vi "pigeon_ver4_1.vi"() -> ()   [LabVIEW 2016]
uses:
  <vilib>/Platform/TimedLoop/XDataNode/timing_clust.ctl
  <vilib>/Platform/TimedLoop/XDataNode/nitl_modes.ctl
  <vilib>/Platform/TimedLoop/XDataNode/wakeup.ctl
  <vilib>/rvi/Emulation/niFpgaGetClockAttributes.vi
  <vilib>/rvi/Emulation/niFpgaSctlEmulationGetInTimedLoop.vi
  <vilib>/rvi/Emulation/niFpgaEmulationReportErrorSimple.vi
  <vilib>/rvi/eio/common/nirviEmuTemplateMethod_errors.vi
  <vilib>/rvi/Emulation/niFpgaProcessEmulError.vi
  <vilib>/rvi/Emulation/niFpgaCriticalErrorInLSC.vi
  <vilib>/rvi/Memory/Memory_Emulation/nirvimemoryFastEmulation.vi
  <vilib>/rvi/Memory/Memory_Emulation/nirvimemoryEmulation.vi
  <vilib>/rvi/Emulation/niFpgaEmulationIsFPGAContextNoSignature.vi
  <vilib>/rvi/DataTransferAndStorage/Container/Common/niFpgaContainerGetUniqueNameForEmu.vi
  <vilib>/rvi/errors/nirviReportUnexpectedCaseInternalError (U32).vi
  <vilib>/rvi/interface/RandomDataEmulation/niFpgaRandomDataHandleErrors.vi
  <vilib>/eio/EIONode/EIONode.xnode
  <vilib>/Platform/TimedLoop/XDataNode/XDataNode.xnode
  <vilib>/rvi/DataTransferAndStorage/Container/XNode/niFpgaContainer.xnode
  <vilib>/rvi/interface/RandomDataEmulation/nirviRandomDataFpgaReadWriteTemplate.vi
  <vilib>/Platform/TimedLoop/XDataNode/XDNodeRunTimeDep.lvlib
panel:
  in  "AO5":i16
  out "AI2":i16
  in  "Tab Control":enum32{"pigeon"}(tab)
  out "trigger AI1":bool
  in  "Tab Control 2":enum32{"square wave generator 1", "coils"}(tab)
  in  "square wave  on?":bool
  in  "square wave period":i32
  in  "IGBTswitch":bool caption="IGBT Switch circular"
  in  "Manual Override":bool
  in  "circular coil current":i16(slide) scale=0.0..32768.0
  out "FIFO size":i16
  in  "AO0":i16
  in  "AO1":i16
  in  "AO2":i16
  in  "Run program":bool
  in  "halt processor":bool
  out "control flags":i8 format="%b"
  in  "host operation":i16
  in  "address":u16
  in  "data1":u16
  in  "data2":i32
  in  "repeat program":i32
  out "IP address":i16
  out "PMT1":i16=-4740
  out "ReA":i32
  out "RegB":i16
  out "RegC":i16
  out "exttrigger":bool=TRUE
  out "AI1":i16=161
  out "RegD":i16
  in  "AO4":i16
  in  "AO3":i16
  out "Connector0/AI0":i16
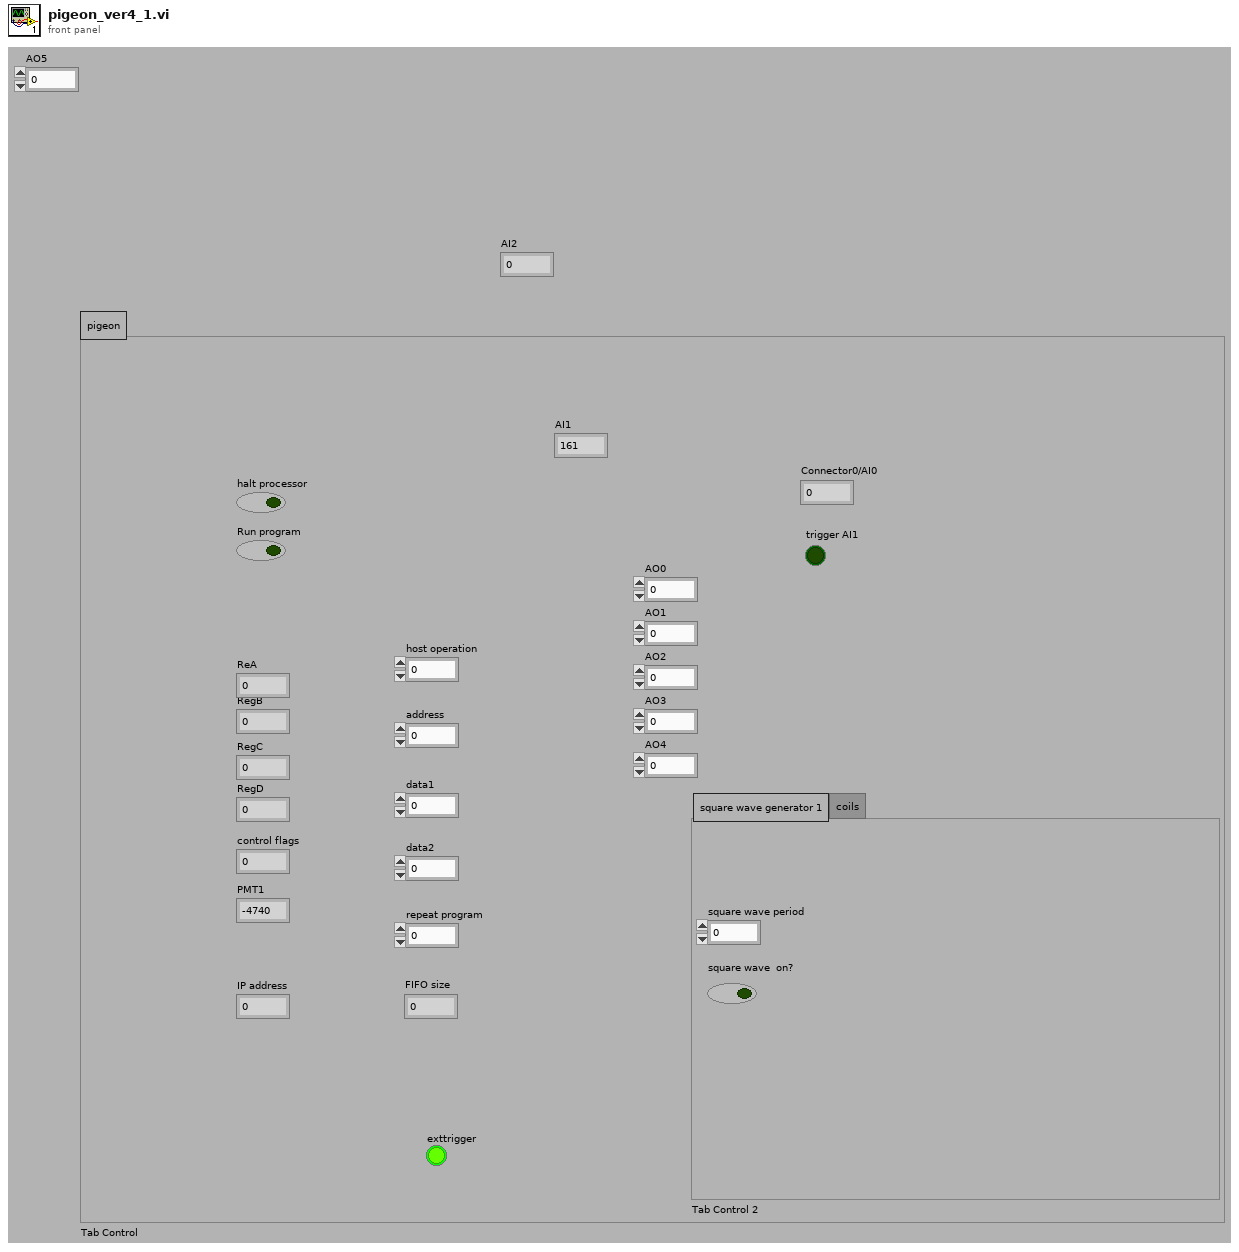
[diagram p1: front panel]
types:
  T1 = typedef "XDNodeRunTimeDep.lvlib/timing_clust.ctl" = cluster{"Expected End [f-1]":u64, "Actual End [f-1]":u64, "Finished Late? [f-1]":bool, "Expected End [i-1]":u64, "Actual End [i-1]":u64, "Finished Late? [i-1]":bool, "Expected Start [i]":u64, "Actual Start [i]":u64, "Expected Start [f]":u64, "Actual Start [f]":u64, "Source Name":string, "Structure Name":string, "Period":i64, "Deadline":i64, "Offset":i64, "Start":i64, "Priority":i32, "Timeout":i32, "Mode":T2, "Wakeup Reason":T3, "Error":errorcluster, "Source Type":string, "Secondary Source Type":string, "Global End Time":u64, "Global Start Time":u64, "Frame Duration":u64, "Iteration Duration":u64, "Assigned CPU":i32, "I/O Scan Engine Mode":u32}
  T2 = typedef "XDNodeRunTimeDep.lvlib/nitl_modes.ctl" = enum32{"No Change", "Process missed periods, maintain original phase", "Discard missed periods, maintain original phase", "Process missed periods, ignore original phase", "Discard missed periods, ignore original phase"}
  T3 = typedef "XDNodeRunTimeDep.lvlib/wakeup.ctl" = enum32{"Normal", "Aborted", "Asynchronous wakeup", "Timing source error", "Timed loop error", "Timeout"}
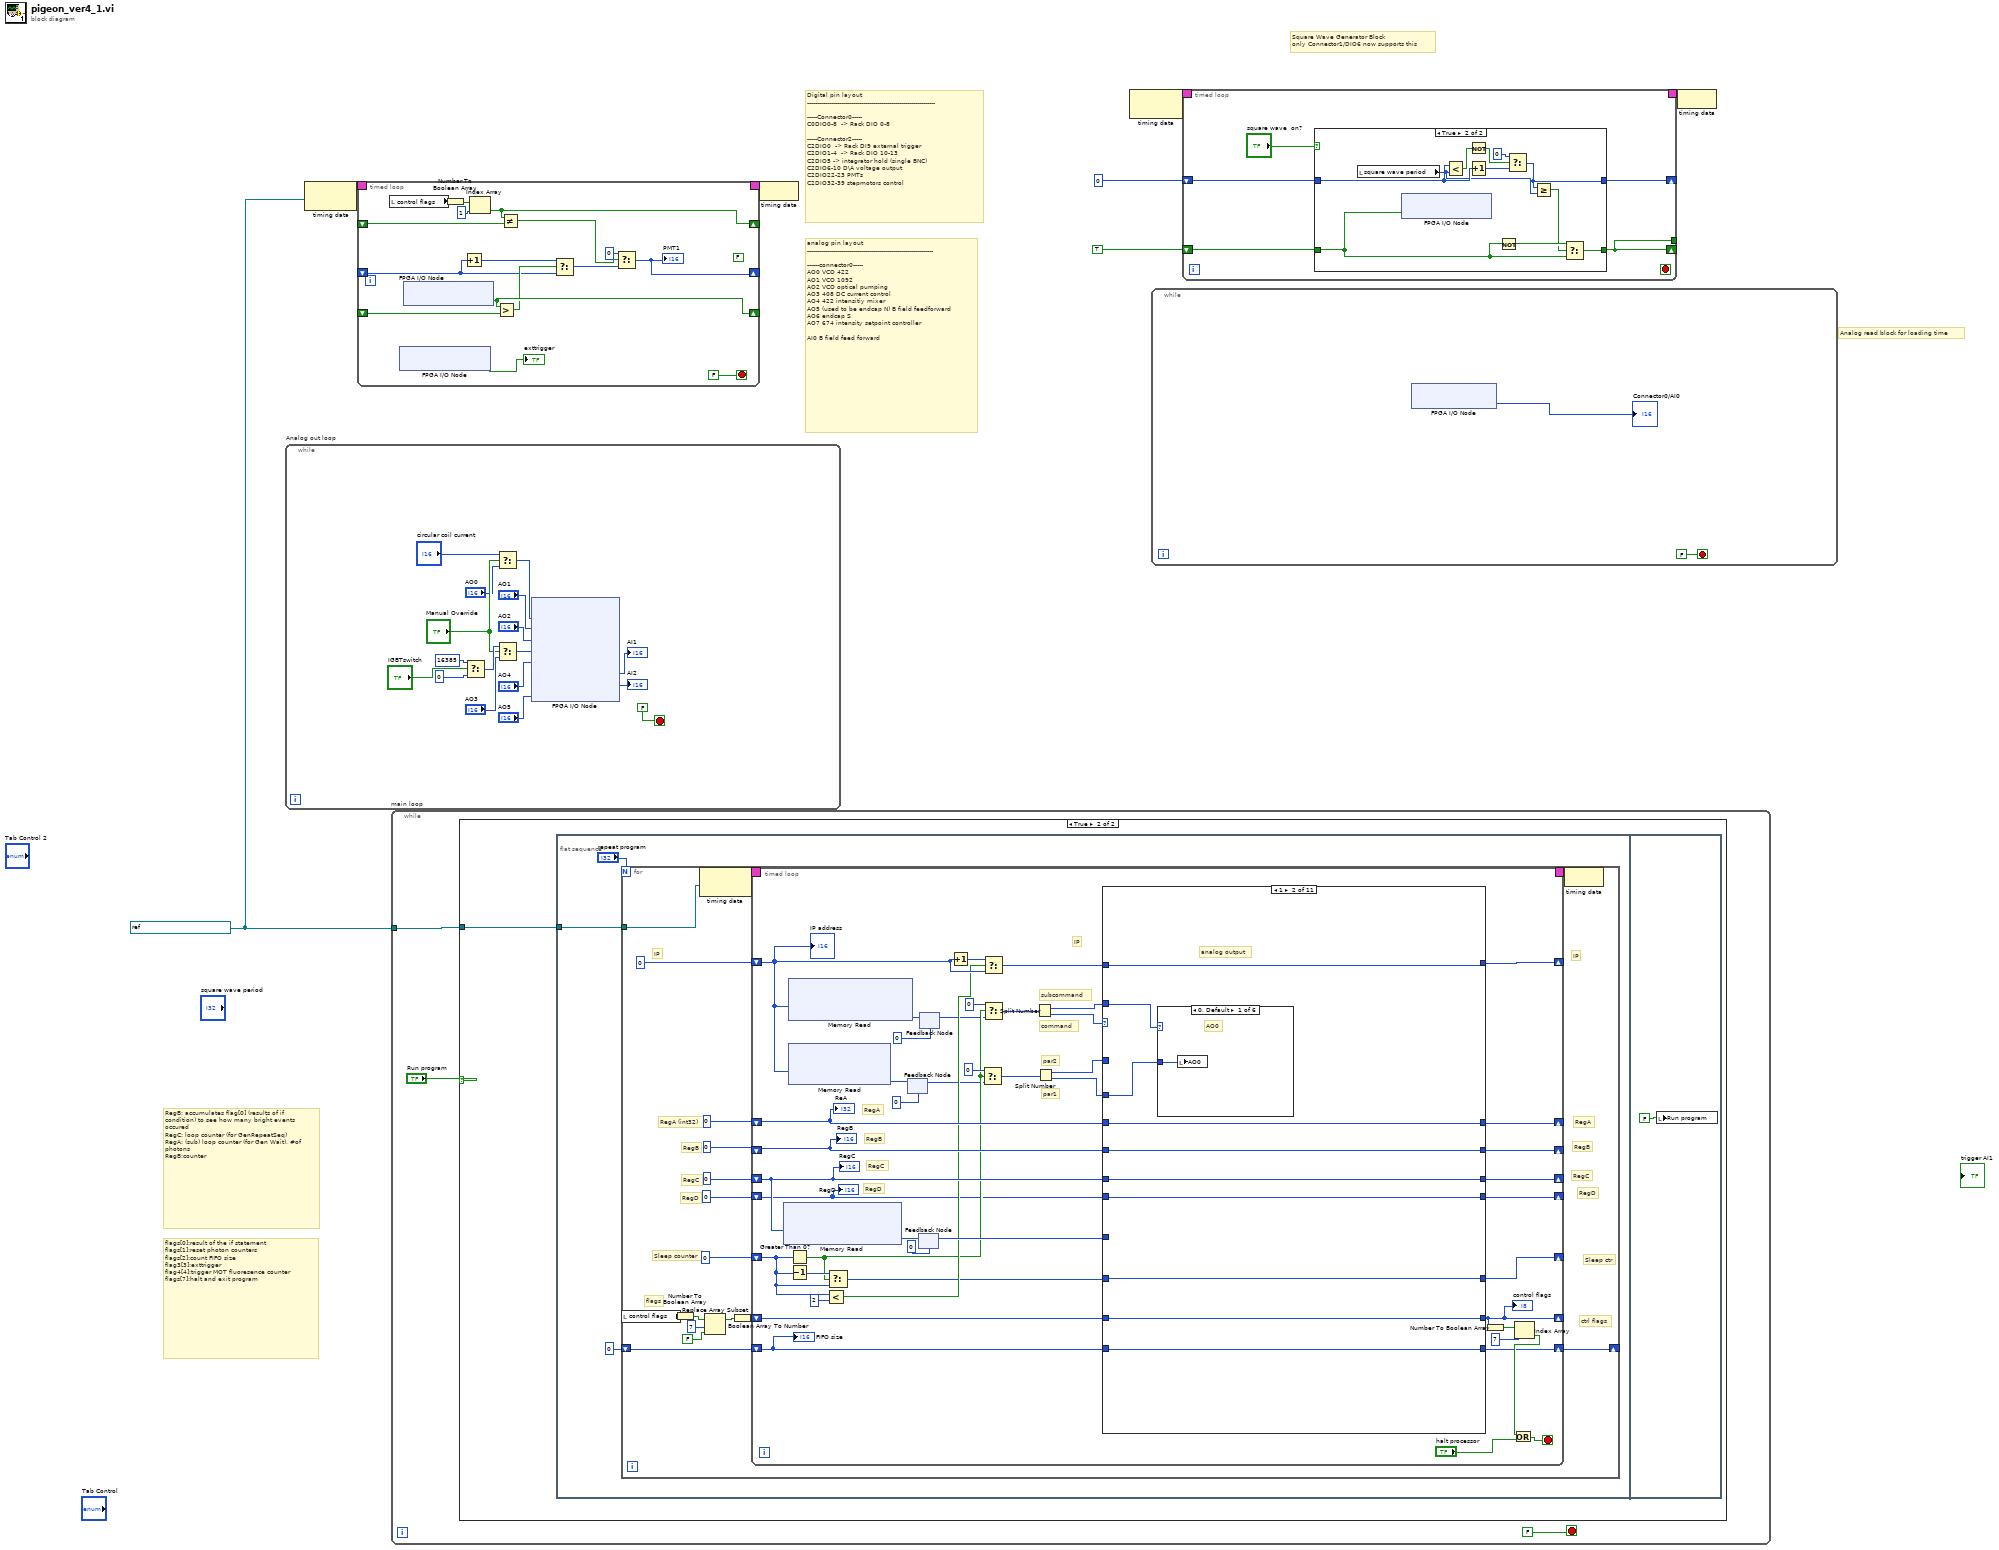
[diagram p0: block diagram]
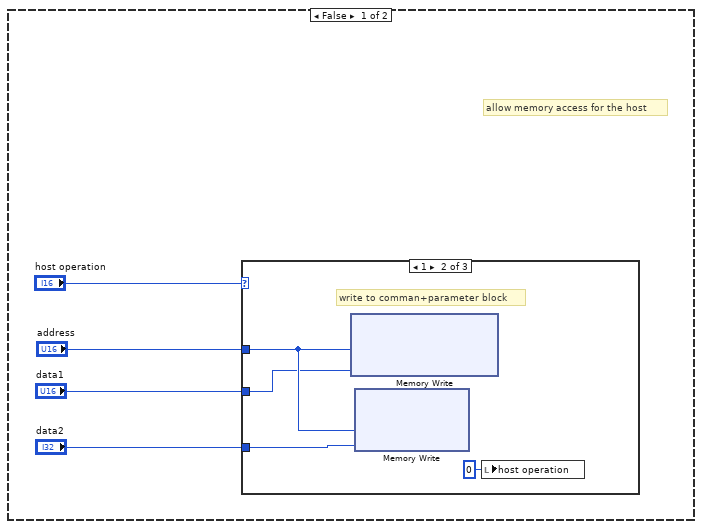
[diagram p3: hidden frame]
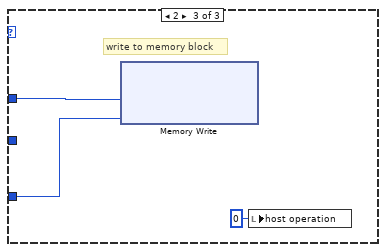
[diagram p5: hidden frame]
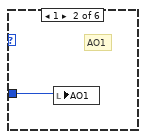
[diagram p7: hidden frame]
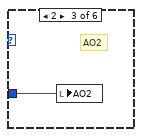
[diagram p8: hidden frame]
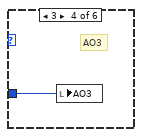
[diagram p9: hidden frame]
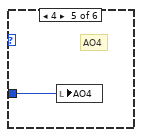
[diagram p10: hidden frame]
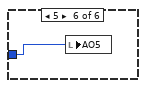
[diagram p11: hidden frame]
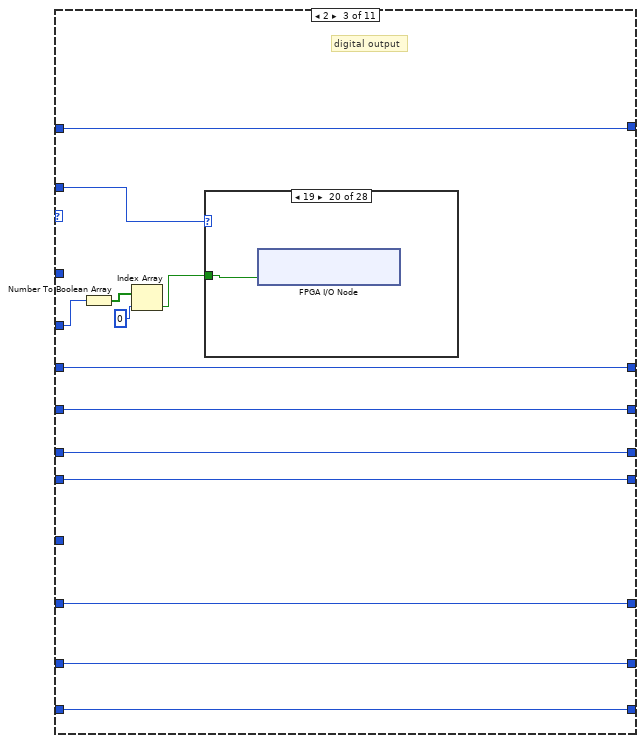
[diagram p12: hidden frame]
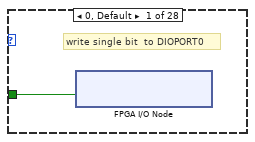
[diagram p13: hidden frame]
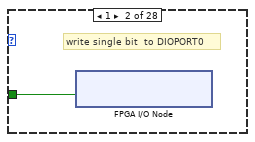
[diagram p14: hidden frame]
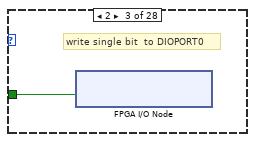
[diagram p15: hidden frame]
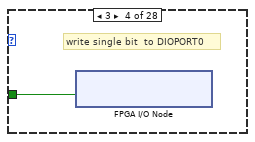
[diagram p16: hidden frame]
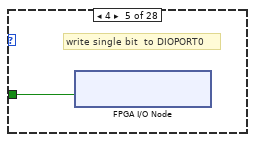
[diagram p17: hidden frame]
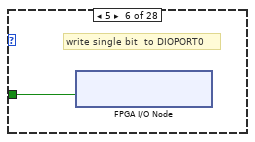
[diagram p18: hidden frame]
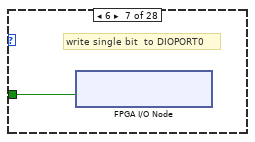
[diagram p19: hidden frame]
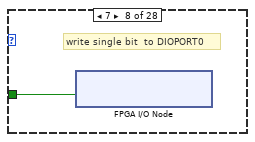
[diagram p20: hidden frame]
diagram:
  w5 = refnum<k21> "40 MHz Onboard Clock" ("FPGA Clock")
  # "Analog read block for loading time"
  # "Square Wave Generator Block\nonly Connector1/DIO6 now supports this"
  # "RegB: accumulates flag[0] (results of if condition) to see how many bright events occured\nRegC: loop counter (for GenRepeatSeq)\nRegA: (sub) loop counter (for Gen Wait), #of     photons \nRegB:counter"
  # "flags[0]:result of the if statement\nflags[1]:reset photon counters\nflags[2]:count FIFO size\nflag3[3]:exttrigger\nflag4[4]:trigger MOT fluoresence counter\nflags[7]:halt and exit program"
  # "Digital pin layout\n----------------------------------------------------------------\n\n-----Connector0-----\nC0DIO0-8  -> Rack DIO 0-8\n\n-----Connector2-----\nC2DIO0  -> Rack DI9 external trigger \nC2DIO1-4  -> Rack DIO 10-13\nC2DIO5 -> integrator hold (single BNC)\nC2DIO6-10 D\\A voltage output\nC2DIO22-23 PMTs\nC2DIO32-39 stepmotors control"
  # "analog pin layout\n---------------------------------------------------------------\n\n------connector0-----\nAO0 VCO 422\nAO1 VCO 1092\nAO2 VCO optical pumping\nAO3 408 DC current control\nAO4 422 intensitiy mixer\nAO5 (used to be endcap N) B field feedforward\nAO6 endcap S\nAO7 674 intensity setpoint controller\n\nAI0 B field feed forward"
  n1 = while "Analog out loop" {
    stop <- FALSE stop-if-true
    n2 = Select(t=i16 16385, s="IGBTswitch", f=i16 0) -> (s? t:f=w14:i16)
    n3 = Select(t="circular coil current", s="Manual Override", f="AO0") -> (s? t:f=w8:i16)
    n4 = Select(t=w14, s="Manual Override", f="AO3") -> (s? t:f=w13:i16)
    n5 = xnode "FPGA I/O Node"("Connector0/AO0"=w8, "Connector0/AO1"="AO1", "Connector0/AO2"="AO2", "Connector0/AO3"=w13, "Connector0/AO4"="AO4", "Connector0/AO5"="AO5") -> ("Connector0/AI1"=→"AI1":i16, "Connector0/AI2"=→"AI2":i16)  [unwired: 8 in, 8 out]
  }
  n6 = node-c288(w5) -> (w7:T1)
  n7 = timed-loop {
    timing: w7 -> [_]
    timing-out: [_] -> w6
    shift-right: [w38] -> _
    shift-left: _ -> [w27]
    shift-right: [w31] -> _
    shift-left: _ -> [w40]
    shift-right: [w33] -> _
    shift-left: _ -> [w34]
    stop <- FALSE stop-if-true
    (unwired) FALSE
    n8 = local read "control flags"() -> (w35:i8)
    n9 = xnode "FPGA I/O Node"() -> ("Connector2/DIO0"=→"exttrigger":bool)  [unwired: 1 in, 1 out]
    n10 = xnode "FPGA I/O Node"() -> ("Connector0/DIO0"=w31:bool)  [unwired: 1 in, 1 out]
    n11 = Number To Boolean Array(number=w35) -> (Boolean array=w36:bool[])
    n12 = Increment(x=w27) -> (x+1=w28:u16)
    n13 = Index Array(array=w36, index=1) -> (element=w33:bool)
    n14 = Greater?(x=w31, y=w40) -> (0:w30:bool)
    n15 = Not Equal?(x=w33, y=w34) -> (x != y?=w25:bool)
    n16 = Select(t=w28, s=w30, f=w27) -> (s? t:f=w39:u16)
    n17 = Select(t=u16 0, s=w25, f=w39) -> (s? t:f=w38:u16)
    "PMT1" <- w38
  }
  n18 = while "main loop" {
    tunnel: w5 -> [w43]
    stop <- FALSE ("stop") stop-if-true
    n19 = case shown="True" "Run program" {
      tunnel: w43 -> [_ w57]
      frame False {
        # "allow memory access for the host"
        n20 = case shown="1" "host operation" {
          tunnel: "address" -> [_ w51 w56]
          tunnel: "data1" -> [_ w50 _]
          tunnel: "data2" -> [_ w53 w54]
          frame 0, Default {
          }
          frame 1 {
            # "write to comman+parameter block"
            n21 = xnode ("Memory Write")("Address"=w51, "Data"=w50) -> ()  [unwired: 1 in, 1 out]
            n22 = xnode ("Memory Write")("Address"=w51, "Data"=w53) -> ()  [unwired: 1 in, 1 out]
            n23 = local write "host operation"(i16 0 ("host operation")) -> ()
          }
          frame 2 {
            # "write to memory block"
            n24 = xnode ("Memory Write")("Address"=w56, "Data"=w54) -> ()  [unwired: 1 in, 1 out]
            n25 = local write "host operation"(i16 0 ("host operation")) -> ()
          }
        }
      }
      frame True {
        n26 = flat-sequence {
          tunnel: w57 -> [w59]
          frame #0 {
            n27 = for {
              N: "repeat program" -> [_]
              tunnel: w59 -> [w71]
              shift-right: [w62] -> _
              shift-left: i16 0 -> [w63]
              # "ctrl flags"
              # "Sleep ctr"
              # "RegD"
              # "RegD"
              # "Sleep counter"
              # "flags"
              # "RegC"
              # "RegB"
              # "RegA"
              # "RegC"
              # "RegB"
              # "RegA (int32)"
              # "IP"
              # "IP"
              n28 = local read "control flags"() -> (w66:i8)
              n29 = Number To Boolean Array(number=w66) -> (Boolean array=w70:bool[])
              n30 = node-c288(w71) -> (w77:T1)
              n31 = Replace Array Subset(array=w70, new element=FALSE ("new element/subarray"), index=7) -> (w68:bool[])
              n32 = Boolean Array To Number(Boolean array=w68) -> (number=w69:u8)
              n33 = timed-loop {
                timing: w77 -> [_]
                timing-out: [_] -> w76
                shift-right: [w112] -> _
                shift-left: i16 0 -> [w95]
                shift-right: [w108] -> _
                shift-left: 0 -> [w104]
                shift-right: [w120] -> _
                shift-left: i16 0 -> [w111]
                shift-right: [w119] -> _
                shift-left: i16 0 -> [w103]
                shift-right: [w109] -> _
                shift-left: w69 -> [w110]
                shift-right: [w102] -> _
                shift-left: i16 0 -> [w93]
                shift-right: [w84] -> w62
                shift-left: w63 -> [w83]
                shift-right: [w81] -> _
                shift-left: i16 0 -> [w82]
                stop <- w115 stop-if-true
                # "RegD"
                # "IP"
                # "RegC"
                # "RegB"
                # "RegA"
                # "par1"
                # "par2"
                # "subcommand"
                # "command"
                n34 = xnode ("Memory Read")("Address"=w103) -> ("Data"=w107:i16)  [unwired: 2 in, 2 out]
                n35 = xnode ("Memory Read")("Address"=w95) -> ("Data"=w90:u16)  [unwired: 1 in, 1 out]
                n36 = xnode ("Memory Read")("Address"=w95) -> ("Data"=w86:i32)  [unwired: 1 in, 1 out]
                n37 = Greater Than 0?(x=w93) -> (x > 0?=w88:bool)
                n38 = Decrement(x=w93) -> (x-1=w94:u32)
                n39 = Less?(x=w93, y=u32 2) -> (x < y?=w92:bool)
                n40 = Select(t=w94, s=w88, f=w93) -> (s? t:f=w91:u32)
                n41 = feedback-in #1(w86) -> ()
                n42 = feedback #1(u32 0 ("Data")) -> (w85:u32)
                n43 = feedback-in #2(w107) -> ()
                n44 = feedback #2(0) -> (w106:i32)
                n45 = feedback-in #3(w90) -> ()
                n46 = feedback #3(u16 0 ("Data")) -> (w87:u16)
                n47 = Increment(x=w95) -> (x+1=w96:u16)
                n48 = Select(t=0, s=w88, f=w85) -> (s? t:f=w99:u32)
                n49 = Select(t=w96, s=w92, f=w95) -> (s? t:f=w101:u16)
                n50 = Select(t=u16 0, s=w88, f=w87) -> (s? t:f=w100:u16)
                n51 = Split Number(x=w100) -> (hi(x)=w121:u8, lo(x)=w122:u8)
                n52 = Split Number(x=w99) -> (hi(x)=w113:u16, lo(x)=w114:u16)
                n53 = case shown="1" w122 {
                  tunnel: w114 -> [_ w139 w151 _ w231 w351 w425 _ _ w484 _]
                  tunnel: w113 -> [_ _ _ _ w224 w350 w424 _ _ w485 _]
                  tunnel: w121 -> [_ w140 w159 w198 w232 w355 _ w443 _ w467 _]
                  tunnel: w104 -> [w130 w138 w158 w190 w230 w352 w429 w447 w463 w483 w502]
                  tunnel: [w130 w138 w158 w190 w227 w352 w429 w447 w463 w482 w502] -> w108
                  tunnel: w111 -> [w129 w137 w157 w189 w229 w353 w430 w446 w466 w481 w503]
                  tunnel: w103 -> [w128 w136 w156 w196 w228 w354 w431 w445 w465 w479 w504]
                  tunnel: [w129 w137 w157 w188 w226 w353 w430 w446 w466 w480 w503] -> w120
                  tunnel: [w128 w136 w156 w196 w225 w354 w431 w445 w465 w478 w504] -> w119
                  tunnel: [w126 w135 w155 w197 w220 w358 w423 w449 w464 w468 w501] -> w112
                  tunnel: w101 -> [w126 w135 w155 w197 w221 w358 _ w449 w464 w469 w501]
                  tunnel: [w127 w134 w154 w194 w222 w357 w422 w438 w460 w472 w507] -> w109
                  tunnel: w110 -> [w127 w134 w154 w195 w223 w356 w422 w437 w459 w473 w507]
                  tunnel: w106 -> [_ _ _ _ w214 w349 _ _ _ _ _]
                  tunnel: w91 -> [w125 w133 w149 w193 w219 w348 w421 w435 w456 w475 w508]
                  tunnel: [w125 w133 w149 w193 w218 w348 w421 w435 w456 w474 w508] -> w102
                  tunnel: w83 -> [w124 w132 w148 w192 w217 w347 w420 w434 w455 w470 w506]
                  tunnel: [w124 w132 w148 w192 w217 w347 w420 w433 w455 w471 w506] -> w84
                  tunnel: w82 -> [w123 w131 w147 w191 w216 w346 w419 w432 w454 w477 w505]
                  tunnel: [w123 w131 w147 w191 w215 w346 w419 w432 w454 w476 w505] -> w81
                  frame 0, Default {
                  }
                  frame 1 {
                    # "analog output"
                    n54 = case shown="0, Default" w140 {
                      tunnel: w139 -> [w141 w142 w143 w144 w145 w146]
                      frame 0, Default {
                        # "AO0"
                        n55 = local write "AO0"(w141) -> ()
                      }
                      frame 1 {
                        # "AO1"
                        n56 = local write "AO1"(w142) -> ()
                      }
                      frame 2 {
                        # "AO2"
                        n57 = local write "AO2"(w143) -> ()
                      }
                      frame 3 {
                        # "AO3"
                        n58 = local write "AO3"(w144) -> ()
                      }
                      frame 4 {
                        # "AO4"
                        n59 = local write "AO4"(w145) -> ()
                      }
                      frame 5 {
                        n60 = local write "AO5"(w146) -> ()
                      }
                    }
                  }
                  frame 2 {
                    # "digital output"
                    n61 = Number To Boolean Array(number=w151) -> (Boolean array=w152:bool[])
                    n62 = Index Array(array=w152, index=0) -> (element=w150:bool)
                    n63 = case shown="19" w159 {
                      tunnel: w150 -> [w160 w161 w162 w163 w164 w165 w166 w167 w168 w169 w170 w171 w172 w173 w174 w175 w176 w177 w178 w179 w180 w181 w182 w183 w184 w185 w186 w187]
                      frame 0, Default {
                        # "write single bit  to DIOPORT0"
                        n64 = xnode "FPGA I/O Node"("Connector1/DIO0"=w160) -> ()  [unwired: 1 in, 1 out]
                      }
                      frame 1 {
                        # "write single bit  to DIOPORT0"
                        n65 = xnode "FPGA I/O Node"("Connector1/DIO1"=w161) -> ()  [unwired: 1 in, 1 out]
                      }
                      frame 2 {
                        # "write single bit  to DIOPORT0"
                        n66 = xnode "FPGA I/O Node"("Connector1/DIO2"=w162) -> ()  [unwired: 1 in, 1 out]
                      }
                      frame 3 {
                        # "write single bit  to DIOPORT0"
                        n67 = xnode "FPGA I/O Node"("Connector1/DIO3"=w163) -> ()  [unwired: 1 in, 1 out]
                      }
                      frame 4 {
                        # "write single bit  to DIOPORT0"
                        n68 = xnode "FPGA I/O Node"("Connector1/DIO4"=w164) -> ()  [unwired: 1 in, 1 out]
                      }
                      frame 5 {
                        # "write single bit  to DIOPORT0"
                        n69 = xnode "FPGA I/O Node"("Connector1/DIO5"=w165) -> ()  [unwired: 1 in, 1 out]
                      }
                      frame 6 {
                        # "write single bit  to DIOPORT0"
                        n70 = xnode "FPGA I/O Node"("Connector1/DIO6"=w166) -> ()  [unwired: 1 in, 1 out]
                      }
                      frame 7 {
                        # "write single bit  to DIOPORT0"
                        n71 = xnode "FPGA I/O Node"("Connector1/DIO7"=w167) -> ()  [unwired: 1 in, 1 out]
                      }
                      frame 8 {
                        # "write single bit  to DIOPORT0"
                        n72 = xnode "FPGA I/O Node"("Connector1/DIO8"=w168) -> ()  [unwired: 1 in, 1 out]
                      }
                      frame 9 {
                        n73 = xnode "FPGA I/O Node"("Connector1/DIO9"=w169) -> ()  [unwired: 1 in, 1 out]
                      }
                      frame 10 {
                        n74 = xnode "FPGA I/O Node"("Connector1/DIO10"=w170) -> ()  [unwired: 1 in, 1 out]
                      }
                      frame 11 {
                        n75 = xnode "FPGA I/O Node"("Connector1/DIO11"=w171) -> ()  [unwired: 1 in, 1 out]
                      }
                      frame 12 {
                        n76 = xnode "FPGA I/O Node"("Connector1/DIO12"=w172) -> ()  [unwired: 1 in, 1 out]
                      }
                      frame 13 {
                        n77 = xnode "FPGA I/O Node"("Connector1/DIO13"=w173) -> ()  [unwired: 1 in, 1 out]
                      }
                      frame 14 {
                        n78 = xnode "FPGA I/O Node"("Connector1/DIO14"=w174) -> ()  [unwired: 1 in, 1 out]
                      }
                      frame 15 {
                        n79 = xnode "FPGA I/O Node"("Connector1/DIO15"=w175) -> ()  [unwired: 1 in, 1 out]
                      }
                      frame 16 {
                        n80 = xnode "FPGA I/O Node"("Connector1/DIO16"=w176) -> ()  [unwired: 1 in, 1 out]
                      }
                      frame 17 {
                        n81 = xnode "FPGA I/O Node"("Connector1/DIO17"=w177) -> ()  [unwired: 1 in, 1 out]
                      }
                      frame 18 {
                        n82 = xnode "FPGA I/O Node"("Connector1/DIO18"=w178) -> ()  [unwired: 1 in, 1 out]
                      }
                      frame 19 {
                        n83 = xnode "FPGA I/O Node"("Connector1/DIO19"=w179) -> ()  [unwired: 1 in, 1 out]
                      }
                      frame 20 {
                        n84 = xnode "FPGA I/O Node"("Connector2/DIO12"=w180) -> ()  [unwired: 1 in, 1 out]
                      }
                      frame 21 {
                        n85 = xnode "FPGA I/O Node"("Connector2/DIO17"=w181) -> ()  [unwired: 1 in, 1 out]
                      }
                      frame 22 {
                        n86 = xnode "FPGA I/O Node"("Connector2/DIO19"=w182) -> ()  [unwired: 1 in, 1 out]
                      }
                      frame 23 {
                        n87 = xnode "FPGA I/O Node"("Connector2/DIO18"=w183) -> ()  [unwired: 1 in, 1 out]
                      }
                      frame 24 {
                        n88 = xnode "FPGA I/O Node"("Connector2/DIO21"=w184) -> ()  [unwired: 1 in, 1 out]
                      }
                      frame 25 {
                        n89 = xnode "FPGA I/O Node"("Connector2/DIO24"=w185) -> ()  [unwired: 1 in, 1 out]
                      }
                      frame 26 {
                        n90 = xnode "FPGA I/O Node"("Connector2/DIO25"=w186) -> ()  [unwired: 1 in, 1 out]
                      }
                      frame 27 {
                        n91 = xnode "FPGA I/O Node"("Connector2/DIO20"=w187) -> ()  [unwired: 1 in, 1 out]
                      }
                    }
                  }
                  frame 3 {
                    # "photon counting"
                    n92 = case shown="3" w198 {
                      tunnel: [w199 w201 w213] -> w188
                      tunnel: w189 -> [w199 w202 w213]
                      tunnel: w195 -> [w200 w204 w211]
                      tunnel: [w200 w204 w210] -> w194
                      frame 2, Default {
                      }
                      frame 1 {
                        # "PMT1"
                        n93 = local read "PMT1"() -> (w203:i16)
                        n94 = Add(x=w203, y=w202) -> (x+y=w201:u16)
                      }
                      frame 3 {
                        # "Reset  photon counter"
                        # "make a Not gate of flag(1)"
                        n95 = Number To Boolean Array(number=w211) -> (Boolean array=w208:bool[])
                        n96 = Index Array(array=w208, index=1) -> (element=w206:bool)
                        n97 = Not(x=w206) -> (.not. x?=w205:bool)
                        n98 = Replace Array Subset(array=w208, new element=w205, index=1) -> (w209:bool[])
                        n99 = Boolean Array To Number(Boolean array=w209) -> (number=w210:u8)
                      }
                    }
                  }
                  frame 4 {
                    # "registers operation"
                    n100 = case shown="7" w232 {
                      tunnel: w231 -> [w238 w248 w255 _ _ _ _ w297 _ _ w324 w337]
                      tunnel: w230 -> [_ w247 w254 w261 w269 w277 w281 w302 w313 w319 w329 w342]
                      tunnel: w229 -> [w241 _ w253 w260 w271 w276 w289 w301 w312 w315 w327 w340]
                      tunnel: w228 -> [w240 w246 _ w263 w270 _ w282 w300 w311 w318 w328 w341]
                      tunnel: [w237 w247 w254 w261 w268 w277 w281 w302 w313 w319 w329 w342] -> w227
                      tunnel: [w241 w248 w253 w260 w271 w276 w288 w301 w312 w317 w327 w340] -> w226
                      tunnel: [w240 w246 w255 w262 w270 w276 w282 w300 w311 w318 w328 w341] -> w225
                      tunnel: w224 -> [w239 _ _ _ _ _ _ w298 _ _ _ w336]
                      tunnel: w223 -> [w236 w245 w252 w259 w267 w275 w283 w299 w310 w322 w332 w345]
                      tunnel: [w236 w245 w252 w259 w267 w275 w283 w299 w310 w322 w332 w345] -> w222
                      tunnel: w221 -> [w235 w244 w251 w258 w266 w274 w280 w291 w305 w321 w331 w344]
                      tunnel: [w235 w244 w251 w258 w266 w274 w280 w294 w308 w321 w331 w344] -> w220
                      tunnel: w219 -> [w234 w243 w250 w257 w265 w273 w279 _ _ w320 w330 w343]
                      tunnel: [w234 w243 w250 w257 w265 w273 w279 w295 w303 w320 w330 w343] -> w218
                      tunnel: w216 -> [w233 w242 w249 w256 w264 w272 w278 w290 w304 w314 _ w335]
                      tunnel: [w233 w242 w249 w256 w264 w272 w278 w290 w304 w314 w325 w334] -> w215
                      tunnel: w214 -> [_ _ _ _ _ _ _ _ w303 _ _ _]
                      frame 0, Default {
                        # "Set par1,2 to RegA"
                        n101 = Join Numbers(hi=w239, lo=w238) -> ((hi.lo)=w237:u32)
                      }
                      frame 1 {
                        # "Set par1 to RegB"
                      }
                      frame 2 {
                        # "Set par1 to RegC"
                      }
                      frame 3 {
                        # "increase RegC by 1"
                        n102 = Increment(x=w263) -> (x+1=w262:u16)
                      }
                      frame 4 {
                        # "increase RegA by 1"
                        n103 = Increment(x=w269) -> (x+1=w268:u32)
                      }
                      frame 5 {
                        # "Set regC to regB"
                      }
                      frame 6 {
                        # "regB<-regB+flags[0]"
                        n104 = Number To Boolean Array(number=w283) -> (Boolean array=w287:bool[])
                        n105 = Index Array(array=w287, index=0) -> (element=w285:bool)
                        n106 = Boolean To (0,1)(Boolean=w285) -> (0, 1=w284:i16)
                        n107 = Add(x=w284, y=w289) -> (x+y=w288:u16)
                      }
                      frame 7 {
                        # "Sleep counter = [par1 par2]"
                        n108 = Join Numbers(hi=w298, lo=w297) -> ((hi.lo)=w295:u32)
                        n109 = Greater?(x=w295, y=u32 0) -> (0:w293:bool)
                        n110 = Decrement(x=w291) -> (x-1=w292:u16)
                        n111 = Select(t=w292, s=w293, f=w291) -> (s? t:f=w294:u16)
                      }
                      frame 11 {
                        # "Sleep counter =par1* memory Block[RegC]"
                        n112 = Greater?(x=w303, y=u32 0) -> (0:w307:bool)
                        n113 = Decrement(x=w305) -> (x-1=w306:u16)
                        n114 = Select(t=w306, s=w307, f=w305) -> (s? t:f=w308:u16)
                      }
                      frame 8 {
                        # "RegB=RegB+ RegA(lo)"
                        n115 = Split Number(x=w319) -> (lo(x)=w316:u16)  [unwired: 1 out]
                        n116 = Add(x=w316, y=w315) -> (x+y=w317:u16)
                      }
                      frame 9 {
                        # "RegD<-AI1+par1"
                        n117 = To Word Integer(number=w324) -> (16bit integer=w323:i16)
                        n118 = local read "AI1"() -> (w326:i16)
                        n119 = Add(x=w323, y=w326) -> (x+y=w325:i16)
                      }
                      frame 10 {
                        # "RegD<-RegD*2^par1*par2"
                        n120 = To Word Integer(number=w336) -> (16bit integer=w338:i16)
                        n121 = To Word Integer(number=w337) -> (16bit integer=w339:i16)
                        n122 = Multiply(x=w338, y=w335) -> (x*y=w333:i16)
                        n123 = Scale By Power Of 2(n=w339, x=w333) -> (x*2^n=w334:i16)
                      }
                    }
                  }
                  frame 5 {
                    # "If statement"
                    n124 = case shown="4" w355 {
                      tunnel: [w368 w376 w384 w392 w402 w405 w413] -> w357
                      tunnel: w356 -> [w367 w375 w383 w391 w401 w406 w414]
                      tunnel: w350 -> [w361 _ _ _ _ _ _]
                      tunnel: w354 -> [_ _ w379 w386 _ _ _]
                      tunnel: w353 -> [_ w370 _ w385 _ _ _]
                      tunnel: w352 -> [w362 _ _ _ _ w403 w411]
                      tunnel: w351 -> [w360 w369 w378 _ _ w404 _]
                      tunnel: w349 -> [_ _ _ _ _ _ w418]
                      frame 0, Default {
                        # "The if regA =  [par1,par2]"
                        n125 = Number To Boolean Array(number=w367) -> (Boolean array=w365:bool[])
                        n126 = Join Numbers(hi=w361, lo=w360) -> ((hi.lo)=w359:u32)
                        n127 = Equal?(x=w359, y=w362) -> (x = y?=w363:bool)
                        n128 = Replace Array Subset(array=w365, new element=w363, index=0) -> (w364:bool[])
                        n129 = Boolean Array To Number(Boolean array=w364) -> (number=w368:u8)
                      }
                      frame 1 {
                        # "The if  regB >  par1"
                        n130 = Number To Boolean Array(number=w375) -> (Boolean array=w373:bool[])
                        n131 = Greater?(x=w370, y=w369) -> (0:w371:bool)
                        n132 = Replace Array Subset(array=w373, new element=w371, index=0) -> (w372:bool[])
                        n133 = Boolean Array To Number(Boolean array=w372) -> (number=w376:u8)
                      }
                      frame 2 {
                        # "The if  regC=  par1"
                        n134 = Number To Boolean Array(number=w383) -> (Boolean array=w381:bool[])
                        n135 = Equal?(x=w378, y=w379) -> (x = y?=w377:bool)
                        n136 = Replace Array Subset(array=w381, new element=w377, index=0) -> (w380:bool[])
                        n137 = Boolean Array To Number(Boolean array=w380) -> (number=w384:u8)
                      }
                      frame 3 {
                        # "The if  regB> regC"
                        n138 = Number To Boolean Array(number=w391) -> (Boolean array=w389:bool[])
                        n139 = Greater?(x=w385, y=w386) -> (0:w387:bool)
                        n140 = Replace Array Subset(array=w389, new element=w387, index=0) -> (w388:bool[])
                        n141 = Boolean Array To Number(Boolean array=w388) -> (number=w392:u8)
                      }
                      frame 4 {
                        w397 = 3 ("index")
                        # "external trigger rising edge"
                        n142 = Number To Boolean Array(number=w401) -> (Boolean array=w398:bool[])
                        n143 = local read "exttrigger"() -> (w394:bool)
                        n144 = Index Array(array=w398, index=w397) -> (element=w396:bool)
                        n145 = Not(x=w396) -> (.not. x?=w395:bool)
                        n146 = And(x=w394, y=w395) -> (x .and. y?=w393:bool)
                        n147 = Replace Array Subset(array=w398, new element #1=w393, index #1=0 ("index"), new element #2=w394, index #2=w397) -> (w399:bool[])
                        n148 = Boolean Array To Number(Boolean array=w399) -> (number=w402:u8)
                      }
                      frame 5 {
                        # "The if  regA >  par1"
                        n149 = Number To Boolean Array(number=w406) -> (Boolean array=w409:bool[])
                        n150 = Greater?(x=w403, y=w404) -> (0:w407:bool)
                        n151 = Replace Array Subset(array=w409, new element=w407, index=0) -> (w408:bool[])
                        n152 = Boolean Array To Number(Boolean array=w408) -> (number=w405:u8)
                      }
                      frame 6 {
                        # "The if  regA == memoryBlock(regC)"
                        n153 = Number To Boolean Array(number=w414) -> (Boolean array=w416:bool[])
                        n154 = Equal?(x=w411, y=w418) -> (x = y?=w412:bool)
                        n155 = Replace Array Subset(array=w416, new element=w412, index=0) -> (w415:bool[])
                        n156 = Boolean Array To Number(Boolean array=w415) -> (number=w413:u8)
                      }
                    }
                  }
                  frame 6 {
                    # "condition (flags[0]) goto\nuse par1=par2 for normal goto"
                    n157 = Number To Boolean Array(number=w422) -> (Boolean array=w428:bool[])
                    n158 = Index Array(array=w428, index=0) -> (element=w426:bool)
                    n159 = Select(t=w425, s=w426, f=w424) -> (s? t:f=w423:u16)
                  }
                  frame 7 {
                    w436 = 2 ("index")
                    # "make a Not gate of flag(2)"
                    # "push  to FIFO"
                    n160 = case shown="4" w443 {
                      tunnel: w447 -> [w450 _ _ _]
                      tunnel: w446 -> [_ w451 _ _]
                      tunnel: w445 -> [_ _ w452 _]
                      tunnel: [w450 w451 w452 w453] -> w444
                      frame 0, Default {
                        # "push RegA"
                      }
                      frame 1 {
                        # "push RegB"
                      }
                      frame 2 {
                        # "push RegC"
                      }
                      frame 4 {
                        n161 = local read "AI1"() -> (w453:i16)
                      }
                    }
                    n162 = Number To Boolean Array(number=w437) -> (Boolean array=w441:bool[])
                    n163 = Index Array(array=w441, index=w436) -> (element=w440:bool)
                    n164 = Not(x=w440) -> (.not. x?=w439:bool)
                    n165 = Replace Array Subset(array=w441, new element=w439, index=w436) -> (w442:bool[])
                    n166 = Increment(x=w434) -> (x+1=w433:i16)
                    n167 = Boolean Array To Number(Boolean array=w442) -> (number=w438:u8)
                    n168 = xnode ("FIFO Write")("Element"=w444, "Timeout"=0) -> ()  [unwired: 1 in, 2 out]
                  }
                  frame 8 {
                    # "Stop and reset program"
                    n169 = Number To Boolean Array(number=w459) -> (Boolean array=w462:bool[])
                    n170 = Replace Array Subset(array=w462, new element=TRUE ("new element/subarray"), index=7) -> (w461:bool[])
                    n171 = Boolean Array To Number(Boolean array=w461) -> (number=w460:u8)
                  }
                  frame 9 {
                    # "Cold Lab Specific instructions"
                    n172 = case shown="0, Default" w467 {
                      tunnel: w485 -> [w498]
                      tunnel: w484 -> [w497]
                      tunnel: w467 -> [w496]
                      tunnel: w483 -> [w493]
                      tunnel: [w493] -> w482
                      tunnel: w481 -> [w492]
                      tunnel: [w492] -> w480
                      tunnel: w479 -> [w491]
                      tunnel: [w491] -> w478
                      tunnel: w477 -> [w490]
                      tunnel: [w490] -> w476
                      tunnel: w475 -> [w489]
                      tunnel: [w489] -> w474
                      tunnel: w473 -> [w488]
                      tunnel: [w488] -> w472
                      tunnel: [w487] -> w471
                      tunnel: w470 -> [w487]
                      tunnel: w469 -> [w486]
                      tunnel: [w486] -> w468
                      frame 0, Default {
                        # "Run Square wave generator"
                        n173 = Greater?(x=w496, y=u8 0) -> (0:w494:bool)
                        n174 = Join Numbers(hi=w498, lo=w497) -> ((hi.lo)=w499:u32)
                        n175 = local write "square wave  on?"(w494) -> ()
                        n176 = local write "square wave period"(w499) -> ()
                      }
                    }
                  }
                  frame 10 {
                    n177 = local write "trigger AI1"(TRUE) -> ()
                  }
                }
                "control flags" <- w109
                n178 = Number To Boolean Array(number=w109) -> (Boolean array=w118:bool[])
                n179 = Index Array(array=w118, index=7) -> (element=w116:bool)
                n180 = Or(x=w116, y="halt processor") -> (x .or. y?=w115:bool)
                "IP address" <- w95
                "ReA" <- w104
                "RegB" <- w111
                "RegC" <- w103
                "FIFO size" <- w83
                "RegD" <- w82
              }
              n181 = node-c288(w76) -> ()
            }
          }
          frame #1 {
            n182 = local write "Run program"(FALSE ("Run program")) -> ()
          }
        }
      }
    }
  }
  n183 = node-c288(w6) -> ()
  n184 = node-c288() -> (w4:T1)  [unwired: 1 in]
  n185 = while {
    stop <- FALSE stop-if-true
    n186 = xnode "FPGA I/O Node"() -> ("Connector0/AI0"=→"Connector0/AI0":i16)  [unwired: 1 in, 1 out]
  }
  n187 = timed-loop {
    shift-right: [w519] -> _
    shift-left: u64 0 -> [w522]
    shift-right: [w521] -> _
    shift-left: TRUE -> [w520]
    timing: w4 -> [_]
    timing-out: [_] -> w3
    tunnel: [w521] -> _
    stop <- _ stop-if-true
    n188 = case shown="True" "square wave  on?" {
      tunnel: w522 -> [w524 w528]
      tunnel: [w523 w532] -> w521
      tunnel: w520 -> [w523 w531]
      tunnel: [w524 w529] -> w519
      frame False {
      }
      frame True {
        n189 = local read "square wave period"() -> (w527:i32)
        n190 = xnode "FPGA I/O Node"("Connector1/DIO6"=w531) -> ()  [unwired: 1 in, 1 out]
        n191 = Less?(x=w528, y=w527) -> (x < y?=w525:bool)
        n192 = Not(x=w525) -> (.not. x?=w526:bool)
        n193 = Increment(x=w528) -> (x+1=w534:u64)
        n194 = Not(x=w531) -> (.not. x?=w533:bool)
        n195 = Select(t=i16 0, s=w526, f=w534) -> (s? t:f=w529:u64)
        n196 = Greater Or Equal?(x=w529, y=w527) -> (x >= y?=w530:bool)
        n197 = Select(t=w533, s=w530, f=w531) -> (s? t:f=w532:bool)
      }
    }
  }
  n198 = node-c288(w3) -> ()
